vi "write json file.vi"(10 "ActorConfiguration":T1, 11 "File Path":path) -> ()   [LabVIEW 2020, in "Template.lvlib" / "Template.lvclass"]
uses:
  Template.lvclass
  typedefs/actor configuration.ctl
  typedefs/shared actor configuration.ctl
  typedefs/resource config/device configuration cluster.ctl
  typedefs/resource config/single resource cluster.ctl
  465192f6-cf10-4ed9-8c5f-bfc9042509a2.vi
  <vilib>/JDP Science/JSONtext/Variant to JSON Text.vi
  <vilib>/JDP Science/JSONtext/LVClass Serializer/JSONtext LVClass Serializer.lvclass
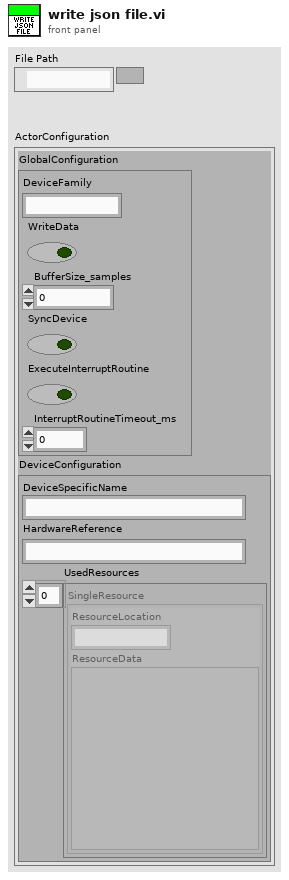
[diagram p1: front panel]
types:
  T1 = typedef "Template.lvlib/Template.lvclass/actor configuration.ctl" = cluster{"GlobalConfiguration":T2, "DeviceConfiguration":T3}
  T2 = typedef "Template.lvlib/Template.lvclass/shared actor configuration.ctl" = cluster{"DeviceFamily":string, "WriteData":bool, "BufferSize_samples":i32, "SyncDevice":bool, "ExecuteInterruptRoutine":bool, "InterruptRoutineTimeout_ms":i32}
  T3 = typedef "Template.lvlib/Template.lvclass/device configuration cluster.ctl" = cluster{"DeviceSpecificName":string, "HardwareReference":string, "UsedResources":T4[]}
  T4 = typedef "Template.lvlib/Template.lvclass/single resource cluster.ctl" = cluster{"ResourceLocation":string, "ResourceData":variant}
  T5 = enum16{"open", "replace", "create", "open or create", "replace or create", "replace or create with confirmation"}
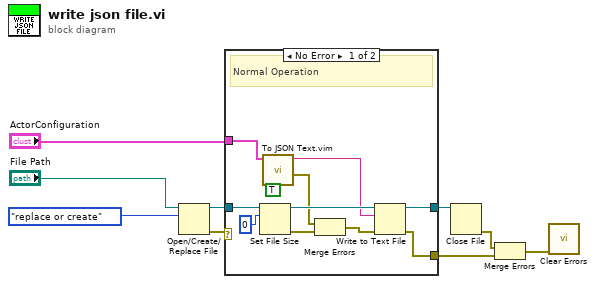
[diagram p0: block diagram]
diagram:
  n1 = Open/Create/Replace File(file path (use dialog)="File Path", operation (0:open)=T5."replace or create") -> (refnum out=w6:refnum<file>, error out=w2:errorcluster)  [unwired: 4 in, 1 out]
  n2 = case shown="No Error" w2 {
    tunnel: w6 -> [w20 w21]
    tunnel: "ActorConfiguration" -> [w10 _]
    tunnel: [w13 w21] -> w7
    tunnel: [w12 _] -> w8
    frame No Error {
      # "Normal Operation"
      n3 = Set File Size(6:i64 0 ("size (in bytes)"), 7:w20) -> (0:w17:errorcluster, 3:w18:refnum<file>)  [unwired: 1 in]
      n4 = call "To JSON Text.vim"("Pretty Print?"=TRUE, "Anything"=w10) -> ("error out"=w14:errorcluster, "<JSON>"=w16:string)  [unwired: 8 in]
      n5 = Merge Errors(w14, w17) -> (w15:errorcluster)
      n6 = Write to Text File(file (use dialog)=w18, text=w16, error in=w15) -> (refnum out=w13:refnum<file>, error out=w12:errorcluster)  [unwired: 1 in, 1 out]
    }
    frame Error {
      # "Errored when opening file"
    }
  }
  n7 = Close File(refnum=w7) -> (error out=w9:errorcluster)  [unwired: 1 in, 1 out]
  n8 = Merge Errors(w9, w8) -> (w1:errorcluster)
  n9 = call <vilib>:"Clear Errors.vi"("error in (no error)"=w1) -> ()  [unwired: 5 in, 2 out]
